vi "Class Tree_Arrow Control.vi"(7 "Direction":enum16{"Down", "Up"}(ring), 8 "error in (no error)":errorcluster, 11 "Tree ref":refnum<vi>) -> (0 "error out":errorcluster, 2 "discard":bool)   [LabVIEW 2023]
doc: "On key up or down, go to next displayed item in list. Assume that keyboard navigation is in use, and replace the last selected item. This will probably fail is multiple items are already selected, and so should be disabled if that's the case."
panel:
  out "first item":bool
  out "last item":bool
  in  "Tree":string[](tree)
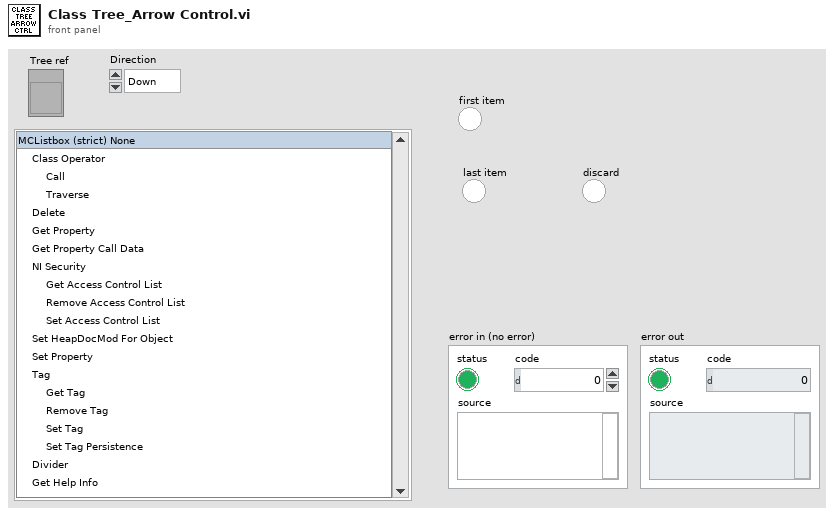
[diagram p1: front panel]
types:
  T1 = enum16{"Unknown", "Base", "Scripting", "Private", "Deprecated", "None", "Divider"}
  T2 = cluster{"Index":u16, "Property Type":enum16{"Unknown", "Base", "Scripting", "Private", "Deprecated", "None", "Divider"}, "ID String":string, "Dotted ID String":string, "Class":string, "Parent":string, "Display name full":string, "Display name short":string, "Parents Array":string[], "Indent":u16}
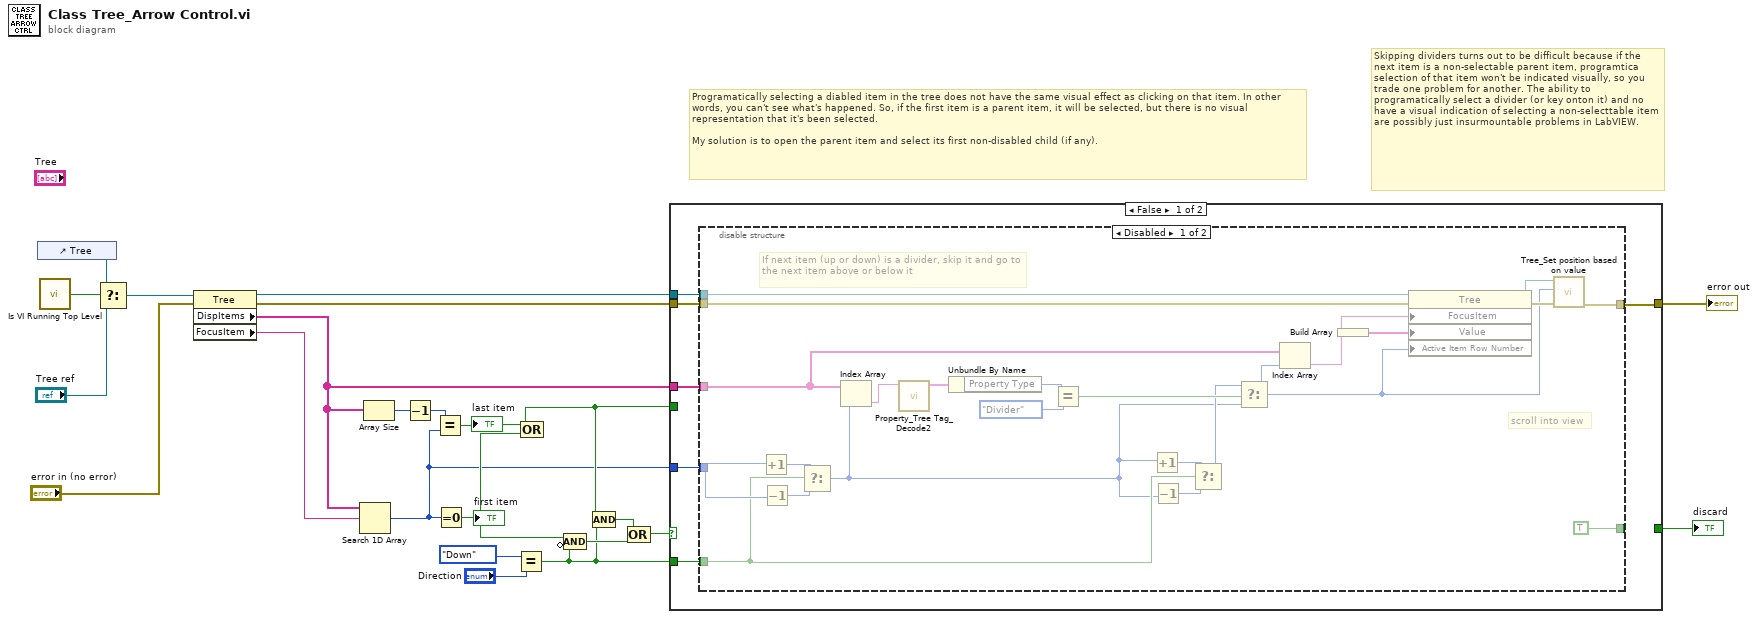
[diagram p0: block diagram]
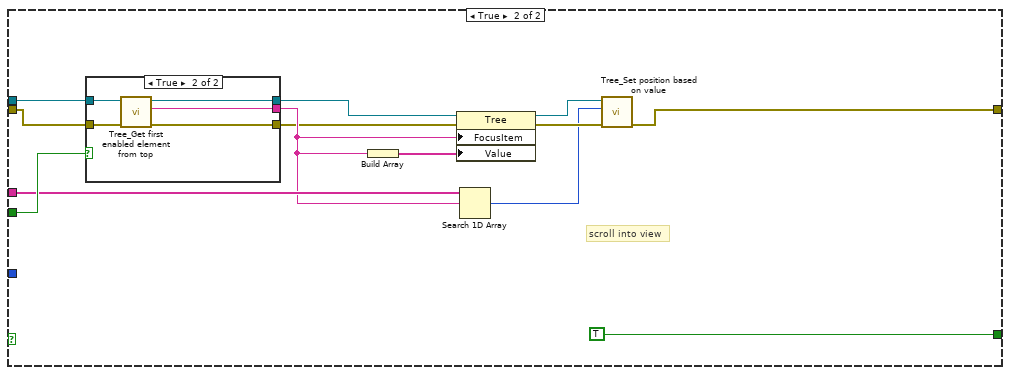
[diagram p3: hidden frame]
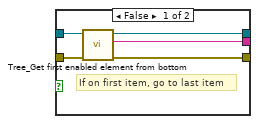
[diagram p4: hidden frame]
diagram:
  # "Skipping dividers turns out to be difficult because if the next item is a non-selectable parent item, programtica selection of that item won't be indicated visually, so you trade one problem for another. The ability to programatically select a divider (or key onton it) and no have a visual indication of selecting a non-selecttable item are possibly just insurmountable problems in LabVIEW."
  # "Programatically selecting a diabled item in the tree does not have the same visual effect as clicking on that item. In other words, you can't see what's happened. So, if the first item is a parent item, it will be selected, but there is no visual representation that it's been selected.\n\nMy solution is to open the parent item and select its first non-disabled child (if any)."
  n1 = control-ref of="Tree"() -> (w22:refnum<vi>)
  n2 = call "Is VI Running Top Level.vi"() -> ("Top Level?"=w18:bool)  [unwired: 5 in]
  n3 = Select(t=w22, s=w18, f="Tree ref") -> (s? t:f=w19:refnum<vi>)
  n4 = property class="Tree"(reference=w19, error in="error in (no error)") -> (reference out=w9:refnum<vi>, error out=w7:errorcluster, "DispItems"=w10:string[], "FocusItem"=w20:string)
  n5 = Search 1D Array(1D array=w10, element=w20) -> (index of element=w2:i32)  [unwired: 1 in]
  n6 = Array Size(array=w10) -> (size(s)=w17:i32)
  n7 = Decrement(x=w17) -> (x-1=w16:i32)
  n8 = Equal?(x=w16, y=w2) -> (x = y?=w15:bool)
  "last item" <- w15
  n9 = Equal To 0?(x=w2) -> (x = 0?=w14:bool)
  "first item" <- w14
  n10 = Equal?(x=enum16{"Down", "Up"}."Down" ("Direction"), y="Direction") -> (x = y?=w1:bool)
  n11 = Compound Arithmetic op=OR(w15, w14) -> ()  [unwired: 1 out]
  n12 = Compound Arithmetic op=AND(w14, invert w1) -> (w12:bool)
  n13 = Compound Arithmetic op=AND(w15, w1) -> (w13:bool)
  n14 = Compound Arithmetic op=OR(w13, w12) -> (w11:bool)
  n15 = case shown="False" w11 {
    tunnel: w10 -> [w26 w63]
    tunnel: w15 -> [_ w64]
    tunnel: w9 -> [w25 w52]
    tunnel: [w23 w59] -> w8
    tunnel: w7 -> [w24 w54]
    tunnel: [_ TRUE ("discard")] -> w5
    tunnel: w2 -> [w28 _]
    tunnel: w1 -> [w27 _]
    frame False {
      n16 = disable-structure shown="Disabled" {
        disable-tunnel: w28 -> [w51 _]
        disable-tunnel: w27 -> [w42 _]
        disable-tunnel: w26 -> [w38 _]
        disable-tunnel: w25 -> [w36 _]
        disable-tunnel: w24 -> [w35 _]
        disable-tunnel: [w31 _] -> w23
        disable-tunnel: [TRUE ("discard") _] -> _
        frame Disabled {
          # "scroll into view"
          # "If next item (up or down) is a divider, skip it and go to the next item above or below it"
          n17 = Increment(x=w51) -> (x+1=w50:i32)
          n18 = Decrement(x=w51) -> (x-1=w49:i32)
          n19 = Select(t=w50, s=w42, f=w49) -> (s? t:f=w39:i32)
          n20 = Index Array(array=w38, index=w39) -> (element=w48:string)
          n21 = call "Property_Tree Tag_Decode2.vi"("Tag In"=w48) -> ("TagData"=w47:T2)  [unwired: 10 in]
          n22 = Unbundle By Name(w47) -> ("Property Type"=w46:T1)
          n23 = Equal?(x=w46, y=T1."Divider" ("Property Type")) -> (x = y?=w41:bool)
          n24 = Increment(x=w39) -> (x+1=w43:i32)
          n25 = Decrement(x=w39) -> (x-1=w44:i32)
          n26 = Select(t=w43, s=w42, f=w44) -> (s? t:f=w40:i32)
          n27 = Select(t=w40, s=w41, f=w39) -> (s? t:f=w29:i32)
          n28 = Index Array(array=w38, index=w29) -> (element=w34:string)
          n29 = Build Array(w34) -> (w37:string[])
          n30 = property class="Tree"(reference=w36, error in=w35, "FocusItem"=w34, "Value"=w37, "Active Item Row Number"=w29) -> (reference out=w32:refnum<vi>, error out=w33:errorcluster)
          n31 = call "Tree_Set position based on value.vi"("error in (no error)"=w33, "Selected Row"=w29, "Tree Ref"=w32) -> ("error out"=w31:errorcluster)  [unwired: 7 in, 1 out]
        }
        frame Enabled {
        }
      }
    }
    frame True {
      # "scroll into view"
      n32 = case shown="True" w64 {
        tunnel: [w65 w71] -> w57
        tunnel: w52 -> [w67 w74]
        tunnel: w54 -> [w69 w73]
        tunnel: [w68 w72] -> w55
        tunnel: [w66 w70] -> w53
        frame False {
          # "If on first item, go to last item"
          n33 = call "Tree_Get first enabled element from bottom.vi"("error in (no error)"=w69, "TreeControl Ref"=w67) -> ("error out"=w68:errorcluster, "First Element Tag"=w65:string, "Tree Control Ref Out"=w66:refnum<vi>)  [unwired: 7 in]
        }
        frame True {
          n34 = call "Tree_Get first enabled element from top.vi"("error in (no error)"=w73, "Tree Control Ref"=w74) -> ("error out"=w72:errorcluster, "First Enabled Element"=w71:string, "Tree Control Ref Out"=w70:refnum<vi>)  [unwired: 7 in]
        }
      }
      n35 = Build Array(w57) -> (w56:string[])
      n36 = property class="Tree"(reference=w53, error in=w55, "FocusItem"=w57, "Value"=w56) -> (reference out=w60:refnum<vi>, error out=w62:errorcluster)
      n37 = Search 1D Array(1D array=w63, element=w57) -> (index of element=w61:i32)  [unwired: 1 in]
      n38 = call "Tree_Set position based on value.vi"("error in (no error)"=w62, "Selected Row"=w61, "Tree Ref"=w60) -> ("error out"=w59:errorcluster)  [unwired: 7 in, 1 out]
    }
  }
  "error out" <- w8
  "discard" <- w5
